vi "Create Limbus Points List.vi"(7 "NoOfPoints":u16=100, 9 "IP Results":T1) -> (1 "Y Points":i16[](array[numeric]), 2 "X Points":i16[](array[numeric]))   [LabVIEW 2015]
uses:
  IP Dev Area/IP results.ctl
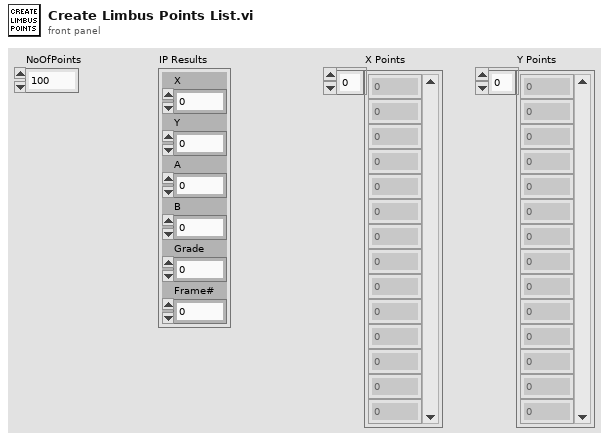
[diagram p1: front panel]
types:
  T1 = typedef "IP results.ctl" = cluster{"X":u16, "Y":u16, "A":dbl, "B":dbl, "Grade":u16, "Frame#":u16}
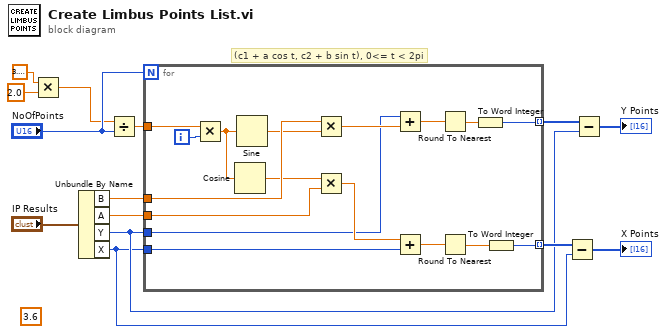
[diagram p0: block diagram]
diagram:
  (unwired) 3.6
  # "(c1 + a cos t, c2 + b sin t), 0<= t < 2pi"
  n1 = Multiply(x=3.141592653589793, y=2.0) -> (x*y=w9:dbl)
  n2 = Unbundle By Name("IP Results") -> ("B"=w6:dbl, "A"=w5:dbl, "Y"=w3:u16, "X"=w1:u16)
  n3 = Divide(x=w9, y="NoOfPoints") -> (x/y=w13:dbl)
  n4 = for {
    N: "NoOfPoints" -> [_]
    tunnel: w3 -> [w26]
    tunnel: w6 -> [w25]
    tunnel: w1 -> [w24]
    tunnel: w5 -> [w23]
    tunnel: w13 -> [w15]
    tunnel: [w18] -> w12 mode=indexing
    tunnel: [w20] -> w7 mode=indexing
    i -> [w22]
    n5 = Multiply(x=w15, y=w22) -> (x*y=w27:dbl)
    n6 = Cosine(x=w27) -> (cos(x)=w16:dbl)
    n7 = Sine(x=w27) -> (sin(x)=w17:dbl)
    n8 = Multiply(x=w25, y=w17) -> (x*y=w31:dbl)
    n9 = Multiply(x=w16, y=w23) -> (x*y=w29:dbl)
    n10 = Add(x=w26, y=w31) -> (x+y=w30:dbl)
    n11 = Add(x=w29, y=w24) -> (x+y=w28:dbl)
    n12 = Round To Nearest(number=w30) -> (nearest integer value=w21:dbl)
    n13 = Round To Nearest(number=w28) -> (nearest integer value=w19:dbl)
    n14 = To Word Integer(number=w21) -> (16bit integer=w20:i16)
    n15 = To Word Integer(number=w19) -> (16bit integer=w18:i16)
  }
  n16 = Subtract(x=w12, y=w1) -> (x-y=→"X Points":u16[])
  n17 = Subtract(x=w7, y=w3) -> (x-y=→"Y Points":u16[])
